vi "FilePaths.vi"(8 "error in":errorcluster) -> (0 "error out":errorcluster, 2 "paths":T1)   [LabVIEW 2014, in "CI Project Builder.lvlib"]
doc: "This VI has the Path to the Classes and the Glyphs, Additional Behavior might be added if you want to load them from a different path. By default they are in Glyphs folder and Classes folder in the main directory"
uses:
  CI Project Builder.lvlib
  Controls/FilePaths.ctl
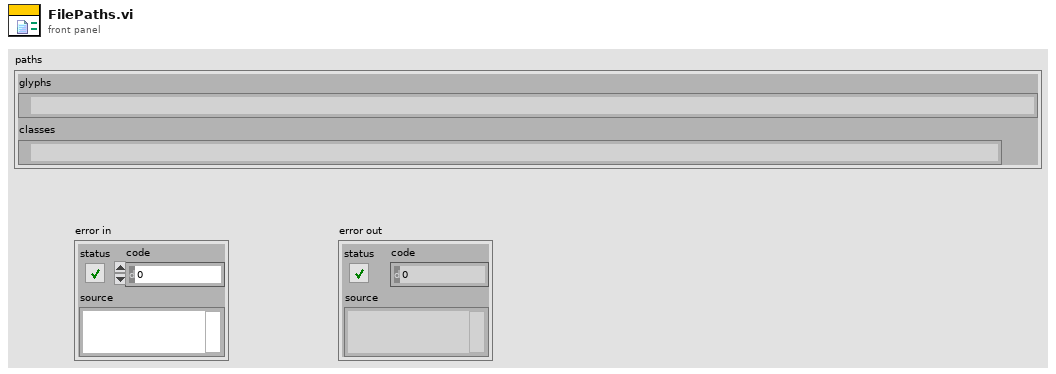
[diagram p1: front panel]
types:
  T1 = typedef "CI Project Builder.lvlib/FilePaths.ctl" = cluster{"glyphs":path, "classes":path}
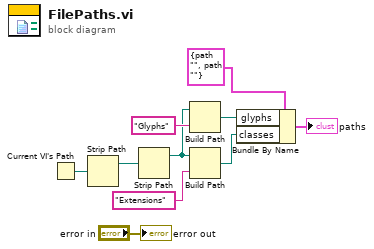
[diagram p0: block diagram]
diagram:
  n1 = Current VI's Path() -> (path=w5:path)
  n2 = Strip Path(path=w5) -> (stripped path=w3:path)  [unwired: 1 out]
  n3 = Strip Path(path=w3) -> (stripped path=w4:path)  [unwired: 1 out]
  n4 = Build Path(base path=w4, name or relative path="Glyphs") -> (appended path=w1:path)
  n5 = Build Path(base path=w4, name or relative path="Extensions") -> (appended path=w2:path)
  n6 = Bundle By Name(cluster=T1 {"glyphs"=path "", "classes"=path ""} ("Cluster 2"), "glyphs"=w1, "classes"=w2) -> (→"paths":T1)
  "error out" <- "error in"
